vi "Read Smooth Segments.vi"(8 "error in (no error)":errorcluster, 11 "Path Settings in":refnum<class "Path Settings.lvclass">) -> (0 "error out":errorcluster, 2 "Smooth Segments":dbl, 3 "Path Settings out":refnum<class "Path Settings.lvclass">)   [LabVIEW 2019, in "Path Settings.lvclass"]
uses:
  Path Settings.lvclass
  Path Settings.lvclass/Path Settings.ctl
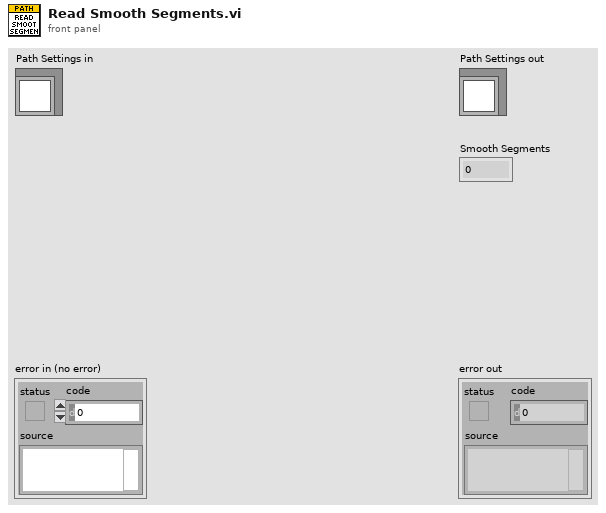
[diagram p1: front panel]
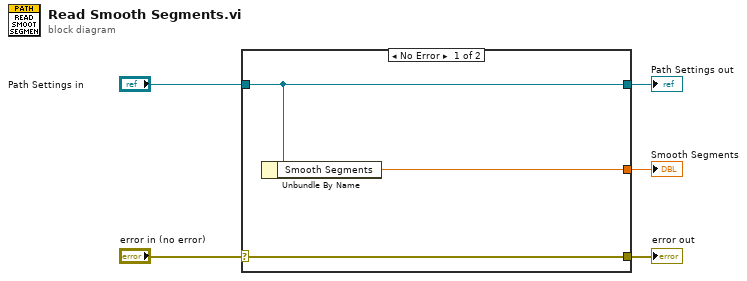
[diagram p0: block diagram]
diagram:
  n1 = case shown="No Error" "error in (no error)" {
    selector: "error in (no error)" -> [w8 w9]
    tunnel: [w8 w9] -> w4
    tunnel: [w7 w10] -> w2
    tunnel: "Path Settings in" -> [w7 w10]
    tunnel: [w6 _] -> w1
    frame No Error {
      n2 = Unbundle By Name(w7) -> ("Smooth Segments"=w6:dbl)
    }
    frame Error {
    }
  }
  "error out" <- w4
  "Path Settings out" <- w2
  "Smooth Segments" <- w1
